vi "Untitled 1.vi"() -> ()   [LabVIEW 2020]
panel:
  in  "New Game":bool
  out "Turno":string
  in  "Ring 42":u16(ring)
  in  "Ring 41":u16(ring)
  in  "Ring 40":u16(ring)
  in  "Ring 39":u16(ring)
  in  "Ring 38":u16(ring)
  in  "Ring 37":u16(ring)
  in  "Ring 36":u16(ring)
  in  "Ring 35":u16(ring)
  in  "Ring 34":u16(ring)
  in  "Ring 33":u16(ring)
  in  "Ring 32":u16(ring)
  in  "Ring 31":u16(ring)
  in  "Ring 30":u16(ring)
  in  "Ring 29":u16(ring)
  in  "Ring 28":u16(ring)
  in  "Ring 27":u16(ring)
  in  "Ring 26":u16(ring)
  in  "Ring 25":u16(ring)
  in  "Ring 24":u16(ring)
  in  "Ring 23":u16(ring)
  in  "Ring 22":u16(ring)
  in  "Ring 21":u16(ring)
  in  "Ring 20":u16(ring)
  in  "Ring 19":u16(ring)
  in  "Ring 18":u16(ring)
  in  "Ring 17":u16(ring)
  in  "Ring 16":u16(ring)
  in  "Ring 15":u16(ring)
  in  "Ring 14":u16(ring)
  in  "Ring 13":u16(ring)
  in  "Ring 12":u16(ring)
  in  "Ring 11":u16(ring)
  in  "Ring 10":u16(ring)
  in  "Ring 9":u16(ring)
  in  "Ring 8":u16(ring)
  in  "Ring 7":u16(ring)
  in  "Ring 6":u16(ring)
  in  "Ring 5":u16(ring)
  in  "Ring 4":u16(ring)
  in  "Ring 3":u16(ring)
  in  "Ring 2":u16(ring)
  in  "Ring":u16(ring)
  # "CUATRO EN LINEA"
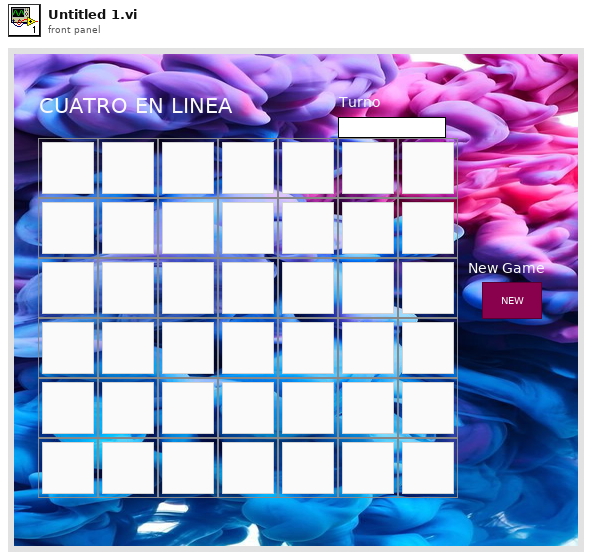
[diagram p1: front panel]
types:
  T1 = typedef "Symbol.ctl" = u16
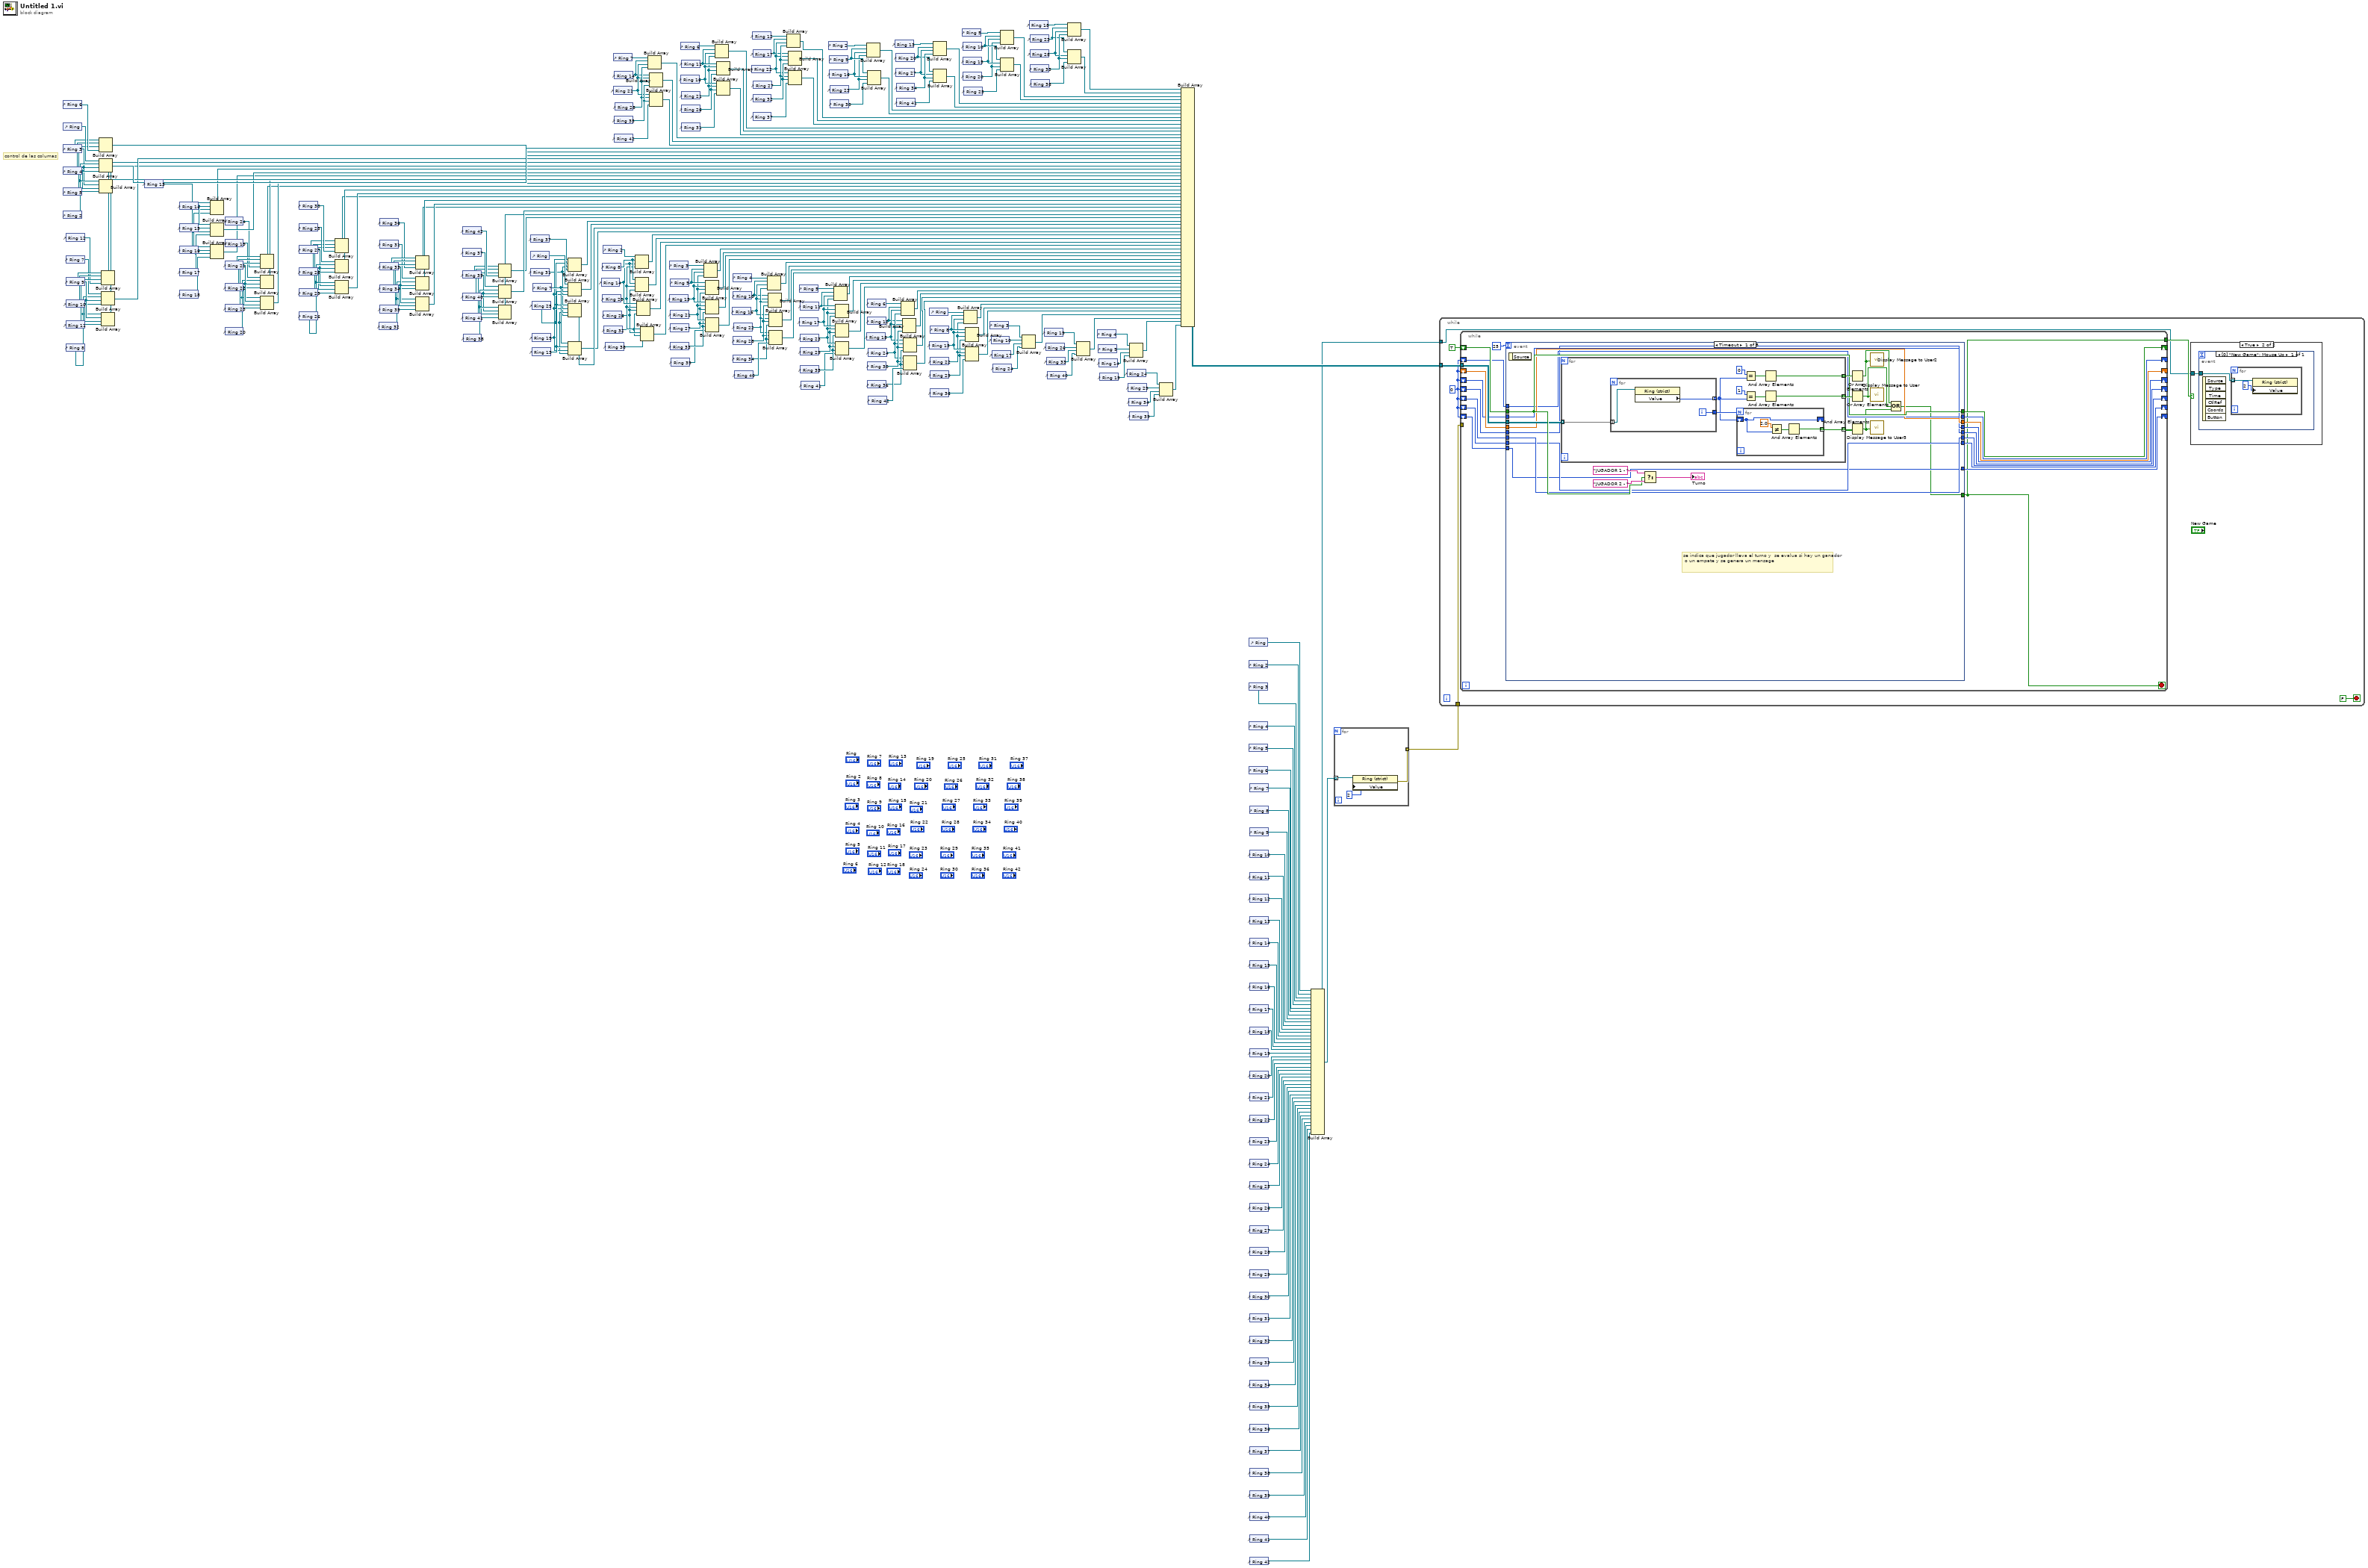
[diagram p0: block diagram]
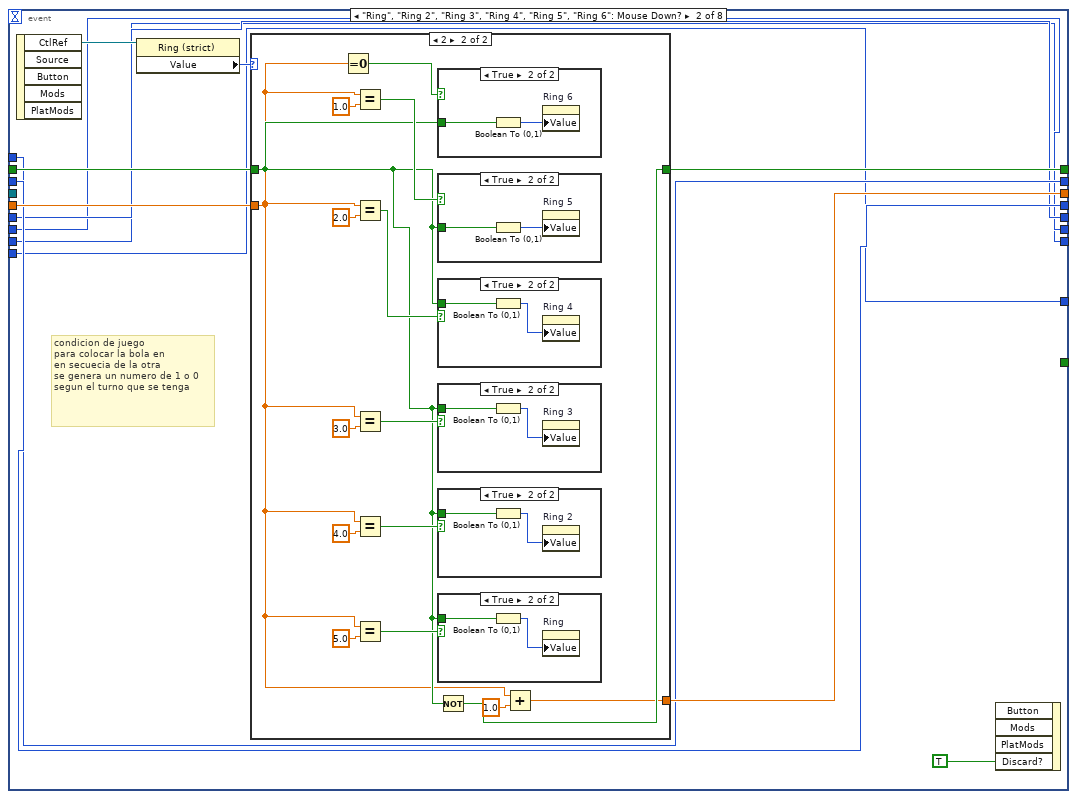
[diagram p3: hidden frame]
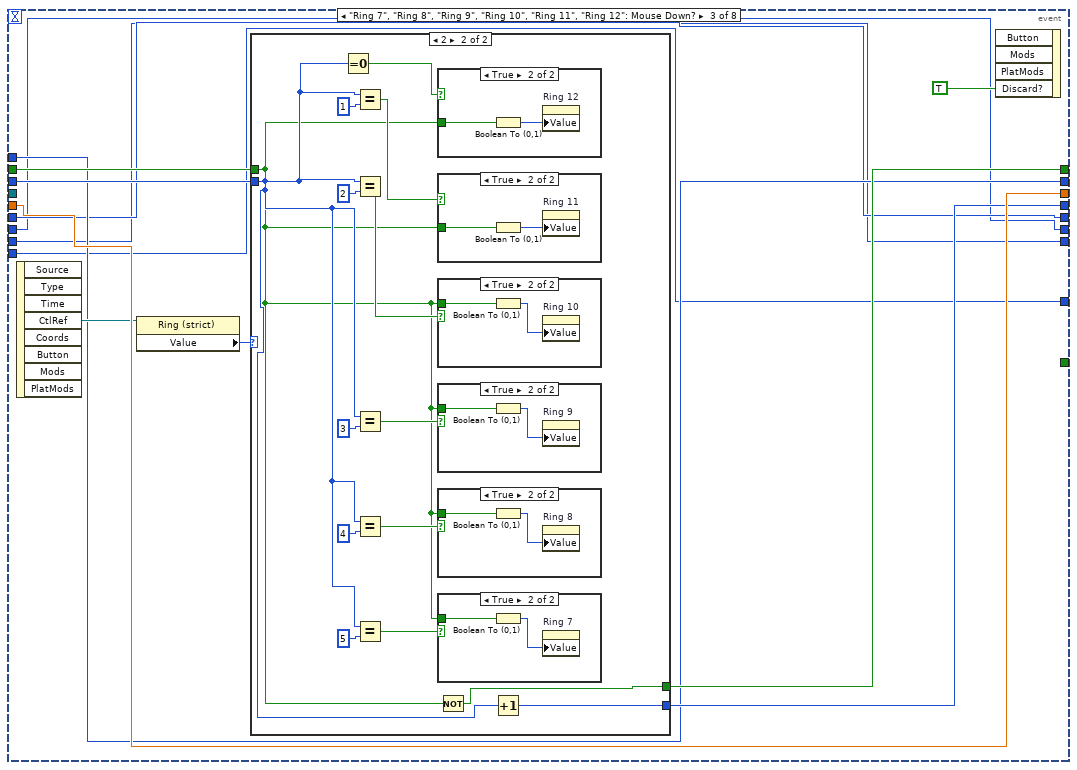
[diagram p11: hidden frame]
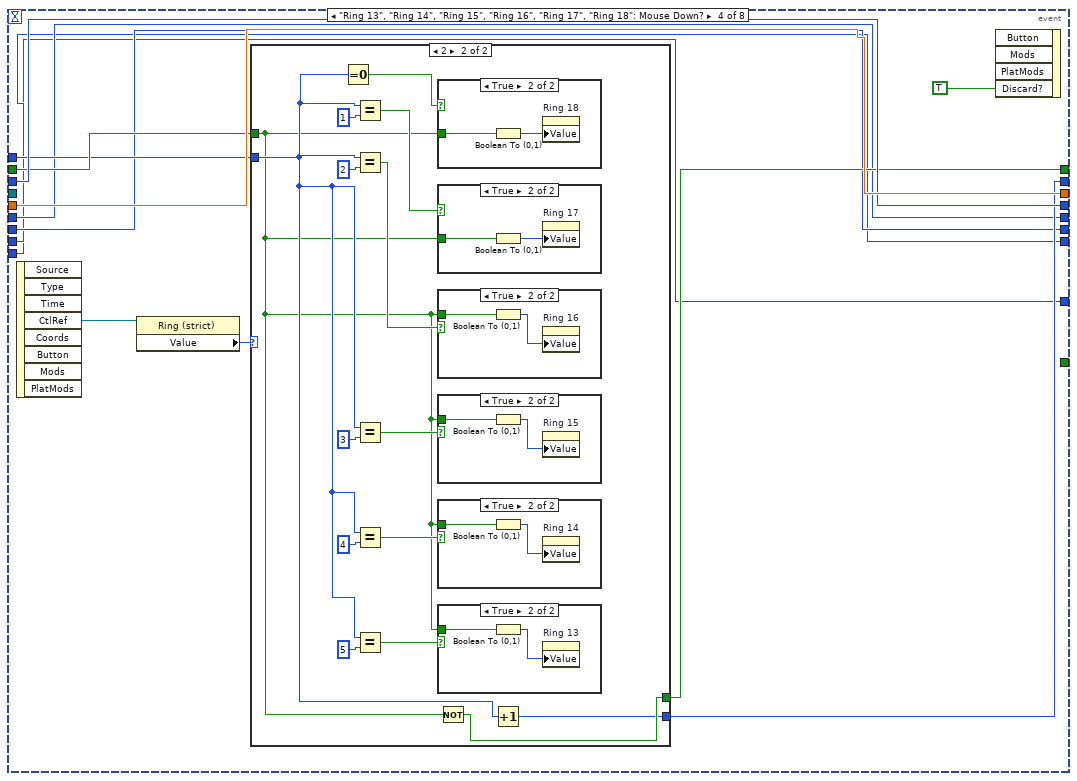
[diagram p19: hidden frame]
diagram:
  # "control de las columas"
  n1 = control-ref of="Ring 6"() -> (w213:refnum<vi>)
  n2 = control-ref of="Ring"() -> (w215:refnum<vi>)
  n3 = control-ref of="Ring 3"() -> (w210:refnum<vi>)
  n4 = control-ref of="Ring 4"() -> (w211:refnum<vi>)
  n5 = control-ref of="Ring 5"() -> (w212:refnum<vi>)
  n6 = control-ref of="Ring 2"() -> (w214:refnum<vi>)
  n7 = control-ref of="Ring 12"() -> (w206:refnum<vi>)
  n8 = control-ref of="Ring 7"() -> (w204:refnum<vi>)
  n9 = control-ref of="Ring 9"() -> (w209:refnum<vi>)
  n10 = control-ref of="Ring 10"() -> (w208:refnum<vi>)
  n11 = control-ref of="Ring 11"() -> (w207:refnum<vi>)
  n12 = control-ref of="Ring 8"() -> (w205:refnum<vi>)
  n13 = Build Array(w210, w211, w212, w213) -> (w201:refnum<vi>[])
  n14 = Build Array(w215, w214, w210, w211) -> (w203:refnum<vi>[])
  n15 = Build Array(w214, w210, w211, w212) -> (w202:refnum<vi>[])
  n16 = Build Array(w209, w208, w207, w206) -> (w198:refnum<vi>[])
  n17 = Build Array(w204, w205, w209, w208) -> (w200:refnum<vi>[])
  n18 = Build Array(w205, w209, w208, w207) -> (w199:refnum<vi>[])
  n19 = control-ref of="Ring 13"() -> (w196:refnum<vi>)
  n20 = control-ref of="Ring 14"() -> (w195:refnum<vi>)
  n21 = control-ref of="Ring 15"() -> (w191:refnum<vi>)
  n22 = control-ref of="Ring 16"() -> (w192:refnum<vi>)
  n23 = control-ref of="Ring 17"() -> (w193:refnum<vi>)
  n24 = control-ref of="Ring 18"() -> (w194:refnum<vi>)
  n25 = Build Array(w196, w195, w191, w192) -> (w190:refnum<vi>[])
  n26 = Build Array(w195, w191, w192, w193) -> (w189:refnum<vi>[])
  n27 = Build Array(w191, w192, w193, w194) -> (w188:refnum<vi>[])
  n28 = control-ref of="Ring 24"() -> (w184:refnum<vi>)
  n29 = control-ref of="Ring 19"() -> (w182:refnum<vi>)
  n30 = control-ref of="Ring 21"() -> (w187:refnum<vi>)
  n31 = control-ref of="Ring 22"() -> (w186:refnum<vi>)
  n32 = control-ref of="Ring 23"() -> (w185:refnum<vi>)
  n33 = control-ref of="Ring 20"() -> (w183:refnum<vi>)
  n34 = Build Array(w187, w186, w185, w184) -> (w179:refnum<vi>[])
  n35 = Build Array(w182, w183, w187, w186) -> (w181:refnum<vi>[])
  n36 = Build Array(w183, w187, w186, w185) -> (w180:refnum<vi>[])
  n37 = control-ref of="Ring 30"() -> (w176:refnum<vi>)
  n38 = control-ref of="Ring 25"() -> (w178:refnum<vi>)
  n39 = control-ref of="Ring 27"() -> (w173:refnum<vi>)
  n40 = control-ref of="Ring 28"() -> (w174:refnum<vi>)
  n41 = control-ref of="Ring 29"() -> (w175:refnum<vi>)
  n42 = control-ref of="Ring 26"() -> (w177:refnum<vi>)
  n43 = Build Array(w173, w174, w175, w176) -> (w170:refnum<vi>[])
  n44 = Build Array(w178, w177, w173, w174) -> (w172:refnum<vi>[])
  n45 = Build Array(w177, w173, w174, w175) -> (w171:refnum<vi>[])
  n46 = control-ref of="Ring 32"() -> (w165:refnum<vi>)
  n47 = control-ref of="Ring 36"() -> (w166:refnum<vi>)
  n48 = control-ref of="Ring 31"() -> (w164:refnum<vi>)
  n49 = control-ref of="Ring 33"() -> (w169:refnum<vi>)
  n50 = control-ref of="Ring 34"() -> (w168:refnum<vi>)
  n51 = control-ref of="Ring 35"() -> (w167:refnum<vi>)
  n52 = Build Array(w169, w168, w167, w166) -> (w161:refnum<vi>[])
  n53 = Build Array(w164, w165, w169, w168) -> (w163:refnum<vi>[])
  n54 = Build Array(w165, w169, w168, w167) -> (w162:refnum<vi>[])
  n55 = control-ref of="Ring 42"() -> (w158:refnum<vi>)
  n56 = control-ref of="Ring 37"() -> (w160:refnum<vi>)
  n57 = control-ref of="Ring 39"() -> (w155:refnum<vi>)
  n58 = control-ref of="Ring 40"() -> (w156:refnum<vi>)
  n59 = control-ref of="Ring 41"() -> (w157:refnum<vi>)
  n60 = control-ref of="Ring 38"() -> (w159:refnum<vi>)
  n61 = Build Array(w155, w156, w157, w158) -> (w152:refnum<vi>[])
  n62 = Build Array(w160, w159, w155, w156) -> (w154:refnum<vi>[])
  n63 = Build Array(w159, w155, w156, w157) -> (w153:refnum<vi>[])
  n64 = control-ref of="Ring 37"() -> (w145:refnum<vi>)
  n65 = control-ref of="Ring"() -> (w151:refnum<vi>)
  n66 = control-ref of="Ring 31"() -> (w146:refnum<vi>)
  n67 = control-ref of="Ring 25"() -> (w147:refnum<vi>)
  n68 = control-ref of="Ring 19"() -> (w148:refnum<vi>)
  n69 = control-ref of="Ring 13"() -> (w149:refnum<vi>)
  n70 = control-ref of="Ring 7"() -> (w150:refnum<vi>)
  n71 = Build Array(w148, w147, w146, w145) -> (w144:refnum<vi>[])
  n72 = Build Array(w151, w150, w149, w148) -> (w143:refnum<vi>[])
  n73 = Build Array(w149, w148, w147, w146) -> (w142:refnum<vi>[])
  n74 = Build Array(w150, w149, w148, w147) -> (w141:refnum<vi>[])
  n75 = control-ref of="Ring 14"() -> (w136:refnum<vi>)
  n76 = control-ref of="Ring 8"() -> (w138:refnum<vi>)
  n77 = control-ref of="Ring 20"() -> (w134:refnum<vi>)
  n78 = control-ref of="Ring 2"() -> (w140:refnum<vi>)
  n79 = control-ref of="Ring 26"() -> (w133:refnum<vi>)
  n80 = control-ref of="Ring 32"() -> (w132:refnum<vi>)
  n81 = control-ref of="Ring 38"() -> (w131:refnum<vi>)
  n82 = control-ref of="Ring 21"() -> (w73:refnum<vi>)
  n83 = control-ref of="Ring 7"() -> (w71:refnum<vi>)
  n84 = control-ref of="Ring 14"() -> (w72:refnum<vi>)
  n85 = control-ref of="Ring 35"() -> (w75:refnum<vi>)
  n86 = control-ref of="Ring 42"() -> (w76:refnum<vi>)
  n87 = control-ref of="Ring 28"() -> (w74:refnum<vi>)
  n88 = Build Array(w140, w138, w136, w134) -> (w139:refnum<vi>[])
  n89 = Build Array(w138, w136, w134, w133) -> (w137:refnum<vi>[])
  n90 = Build Array(w136, w134, w133, w132) -> (w135:refnum<vi>[])
  n91 = Build Array(w134, w133, w132, w131) -> (w130:refnum<vi>[])
  n92 = Build Array(w71, w72, w73, w74) -> (w68:refnum<vi>[])
  n93 = Build Array(w72, w73, w74, w75) -> (w69:refnum<vi>[])
  n94 = Build Array(w73, w74, w75, w76) -> (w70:refnum<vi>[])
  n95 = control-ref of="Ring 15"() -> (w125:refnum<vi>)
  n96 = control-ref of="Ring 3"() -> (w129:refnum<vi>)
  n97 = control-ref of="Ring 9"() -> (w127:refnum<vi>)
  n98 = control-ref of="Ring 27"() -> (w122:refnum<vi>)
  n99 = control-ref of="Ring 33"() -> (w121:refnum<vi>)
  n100 = control-ref of="Ring 21"() -> (w123:refnum<vi>)
  n101 = control-ref of="Ring 39"() -> (w120:refnum<vi>)
  n102 = control-ref of="Ring 16"() -> (w65:refnum<vi>)
  n103 = control-ref of="Ring 6"() -> (w67:refnum<vi>)
  n104 = control-ref of="Ring 11"() -> (w66:refnum<vi>)
  n105 = control-ref of="Ring 26"() -> (w63:refnum<vi>)
  n106 = control-ref of="Ring 31"() -> (w62:refnum<vi>)
  n107 = control-ref of="Ring 21"() -> (w64:refnum<vi>)
  n108 = Build Array(w129, w127, w125, w123) -> (w128:refnum<vi>[])
  n109 = Build Array(w127, w125, w123, w122) -> (w126:refnum<vi>[])
  n110 = Build Array(w125, w123, w122, w121) -> (w124:refnum<vi>[])
  n111 = Build Array(w123, w122, w121, w120) -> (w119:refnum<vi>[])
  n112 = Build Array(w67, w66, w65, w64) -> (w59:refnum<vi>[])
  n113 = Build Array(w66, w65, w64, w63) -> (w60:refnum<vi>[])
  n114 = Build Array(w65, w64, w63, w62) -> (w61:refnum<vi>[])
  n115 = control-ref of="Ring 16"() -> (w114:refnum<vi>)
  n116 = control-ref of="Ring 4"() -> (w112:refnum<vi>)
  n117 = control-ref of="Ring 10"() -> (w113:refnum<vi>)
  n118 = control-ref of="Ring 28"() -> (w116:refnum<vi>)
  n119 = control-ref of="Ring 34"() -> (w117:refnum<vi>)
  n120 = control-ref of="Ring 22"() -> (w115:refnum<vi>)
  n121 = control-ref of="Ring 40"() -> (w118:refnum<vi>)
  n122 = control-ref of="Ring 22"() -> (w55:refnum<vi>)
  n123 = control-ref of="Ring 12"() -> (w53:refnum<vi>)
  n124 = control-ref of="Ring 17"() -> (w54:refnum<vi>)
  n125 = control-ref of="Ring 32"() -> (w57:refnum<vi>)
  n126 = control-ref of="Ring 37"() -> (w58:refnum<vi>)
  n127 = control-ref of="Ring 27"() -> (w56:refnum<vi>)
  n128 = Build Array(w112, w113, w114, w115) -> (w111:refnum<vi>[])
  n129 = Build Array(w113, w114, w115, w116) -> (w110:refnum<vi>[])
  n130 = Build Array(w114, w115, w116, w117) -> (w109:refnum<vi>[])
  n131 = Build Array(w115, w116, w117, w118) -> (w108:refnum<vi>[])
  n132 = Build Array(w53, w54, w55, w56) -> (w50:refnum<vi>[])
  n133 = Build Array(w54, w55, w56, w57) -> (w51:refnum<vi>[])
  n134 = Build Array(w55, w56, w57, w58) -> (w52:refnum<vi>[])
  n135 = control-ref of="Ring 17"() -> (w105:refnum<vi>)
  n136 = control-ref of="Ring 5"() -> (w107:refnum<vi>)
  n137 = control-ref of="Ring 11"() -> (w106:refnum<vi>)
  n138 = control-ref of="Ring 29"() -> (w103:refnum<vi>)
  n139 = control-ref of="Ring 35"() -> (w102:refnum<vi>)
  n140 = control-ref of="Ring 23"() -> (w104:refnum<vi>)
  n141 = control-ref of="Ring 41"() -> (w101:refnum<vi>)
  n142 = control-ref of="Ring 2"() -> (w49:refnum<vi>)
  n143 = control-ref of="Ring 9"() -> (w48:refnum<vi>)
  n144 = control-ref of="Ring 16"() -> (w47:refnum<vi>)
  n145 = control-ref of="Ring 23"() -> (w46:refnum<vi>)
  n146 = control-ref of="Ring 30"() -> (w45:refnum<vi>)
  n147 = Build Array(w107, w106, w105, w104) -> (w100:refnum<vi>[])
  n148 = Build Array(w106, w105, w104, w103) -> (w99:refnum<vi>[])
  n149 = Build Array(w105, w104, w103, w102) -> (w98:refnum<vi>[])
  n150 = Build Array(w104, w103, w102, w101) -> (w97:refnum<vi>[])
  n151 = Build Array(w49, w48, w47, w46) -> (w43:refnum<vi>[])
  n152 = control-ref of="Ring 18"() -> (w92:refnum<vi>)
  n153 = Build Array(w48, w47, w46, w45) -> (w44:refnum<vi>[])
  n154 = control-ref of="Ring 6"() -> (w90:refnum<vi>)
  n155 = control-ref of="Ring 12"() -> (w91:refnum<vi>)
  n156 = control-ref of="Ring 30"() -> (w94:refnum<vi>)
  n157 = control-ref of="Ring 36"() -> (w95:refnum<vi>)
  n158 = control-ref of="Ring 24"() -> (w93:refnum<vi>)
  n159 = control-ref of="Ring 42"() -> (w96:refnum<vi>)
  n160 = control-ref of="Ring 13"() -> (w38:refnum<vi>)
  n161 = control-ref of="Ring 20"() -> (w39:refnum<vi>)
  n162 = control-ref of="Ring 27"() -> (w40:refnum<vi>)
  n163 = control-ref of="Ring 34"() -> (w41:refnum<vi>)
  n164 = control-ref of="Ring 41"() -> (w42:refnum<vi>)
  n165 = Build Array(w90, w91, w92, w93) -> (w89:refnum<vi>[])
  n166 = Build Array(w91, w92, w93, w94) -> (w88:refnum<vi>[])
  n167 = Build Array(w92, w93, w94, w95) -> (w87:refnum<vi>[])
  n168 = Build Array(w93, w94, w95, w96) -> (w86:refnum<vi>[])
  n169 = control-ref of="Ring 15"() -> (w83:refnum<vi>)
  n170 = control-ref of="Ring"() -> (w85:refnum<vi>)
  n171 = control-ref of="Ring 8"() -> (w84:refnum<vi>)
  n172 = control-ref of="Ring 29"() -> (w81:refnum<vi>)
  n173 = control-ref of="Ring 36"() -> (w80:refnum<vi>)
  n174 = control-ref of="Ring 22"() -> (w82:refnum<vi>)
  n175 = Build Array(w38, w39, w40, w41) -> (w36:refnum<vi>[])
  n176 = Build Array(w39, w40, w41, w42) -> (w37:refnum<vi>[])
  n177 = control-ref of="Ring 5"() -> (w35:refnum<vi>)
  n178 = control-ref of="Ring 10"() -> (w34:refnum<vi>)
  n179 = control-ref of="Ring 15"() -> (w33:refnum<vi>)
  n180 = control-ref of="Ring 20"() -> (w32:refnum<vi>)
  n181 = control-ref of="Ring 25"() -> (w31:refnum<vi>)
  n182 = Build Array(w85, w84, w83, w82) -> (w79:refnum<vi>[])
  n183 = Build Array(w84, w83, w82, w81) -> (w78:refnum<vi>[])
  n184 = Build Array(w83, w82, w81, w80) -> (w77:refnum<vi>[])
  n185 = control-ref of="Ring 3"() -> (w21:refnum<vi>)
  n186 = control-ref of="Ring 10"() -> (w20:refnum<vi>)
  n187 = control-ref of="Ring 17"() -> (w19:refnum<vi>)
  n188 = control-ref of="Ring 24"() -> (w18:refnum<vi>)
  n189 = Build Array(w35, w34, w33, w32) -> (w29:refnum<vi>[])
  n190 = Build Array(w34, w33, w32, w31) -> (w30:refnum<vi>[])
  n191 = Build Array(w21, w20, w19, w18) -> (w17:refnum<vi>[])
  n192 = control-ref of="Ring 18"() -> (w24:refnum<vi>)
  n193 = control-ref of="Ring 23"() -> (w25:refnum<vi>)
  n194 = control-ref of="Ring 28"() -> (w26:refnum<vi>)
  n195 = control-ref of="Ring 33"() -> (w27:refnum<vi>)
  n196 = control-ref of="Ring 38"() -> (w28:refnum<vi>)
  n197 = control-ref of="Ring 19"() -> (w13:refnum<vi>)
  n198 = control-ref of="Ring 26"() -> (w14:refnum<vi>)
  n199 = control-ref of="Ring 33"() -> (w15:refnum<vi>)
  n200 = control-ref of="Ring 40"() -> (w16:refnum<vi>)
  n201 = Build Array(w24, w25, w26, w27) -> (w22:refnum<vi>[])
  n202 = Build Array(w25, w26, w27, w28) -> (w23:refnum<vi>[])
  n203 = Build Array(w13, w14, w15, w16) -> (w12:refnum<vi>[])
  n204 = control-ref of="Ring 4"() -> (w11:refnum<vi>)
  n205 = control-ref of="Ring 9"() -> (w10:refnum<vi>)
  n206 = control-ref of="Ring 14"() -> (w9:refnum<vi>)
  n207 = control-ref of="Ring 19"() -> (w8:refnum<vi>)
  n208 = control-ref of="Ring 24"() -> (w3:refnum<vi>)
  n209 = control-ref of="Ring 29"() -> (w4:refnum<vi>)
  n210 = control-ref of="Ring 34"() -> (w5:refnum<vi>)
  n211 = Build Array(w11, w10, w9, w8) -> (w7:refnum<vi>[])
  n212 = control-ref of="Ring 39"() -> (w6:refnum<vi>)
  n213 = Build Array(w3, w4, w5, w6) -> (w2:refnum<vi>[])
  n214 = Build Array(w22, w23, w29, w30, w36, w37, w43, w44, w50, w51, w52, w59, w60, w61, w68, w69, w70, w203, w202, w201, w200, w199, w198, w190, w189, w188, w181, w180, w179, w172, w171, w170, w163, w162, w161, w154, w153, w152, w144, w143, w142, w141, w139, w137, w135, w130, w128, w126, w124, w119, w111, w110, w109, w108, w100, w99, w98, w97, w89, w88, w87, w86, w79, w78, w77, w17, w12, w7, w2) -> (w197:refnum<vi>[][])
  n215 = control-ref of="Ring"() -> (w258:refnum<vi>)
  n216 = control-ref of="Ring 2"() -> (w257:refnum<vi>)
  n217 = control-ref of="Ring 3"() -> (w256:refnum<vi>)
  n218 = control-ref of="Ring 4"() -> (w255:refnum<vi>)
  n219 = control-ref of="Ring 5"() -> (w254:refnum<vi>)
  n220 = control-ref of="Ring 6"() -> (w253:refnum<vi>)
  n221 = control-ref of="Ring 7"() -> (w252:refnum<vi>)
  n222 = control-ref of="Ring 8"() -> (w251:refnum<vi>)
  n223 = control-ref of="Ring 9"() -> (w250:refnum<vi>)
  n224 = control-ref of="Ring 10"() -> (w249:refnum<vi>)
  n225 = control-ref of="Ring 11"() -> (w248:refnum<vi>)
  n226 = control-ref of="Ring 12"() -> (w247:refnum<vi>)
  n227 = control-ref of="Ring 13"() -> (w246:refnum<vi>)
  n228 = control-ref of="Ring 14"() -> (w245:refnum<vi>)
  n229 = control-ref of="Ring 15"() -> (w244:refnum<vi>)
  n230 = control-ref of="Ring 16"() -> (w243:refnum<vi>)
  n231 = control-ref of="Ring 17"() -> (w242:refnum<vi>)
  n232 = control-ref of="Ring 18"() -> (w241:refnum<vi>)
  n233 = control-ref of="Ring 19"() -> (w240:refnum<vi>)
  n234 = control-ref of="Ring 20"() -> (w239:refnum<vi>)
  n235 = control-ref of="Ring 21"() -> (w238:refnum<vi>)
  n236 = control-ref of="Ring 22"() -> (w237:refnum<vi>)
  n237 = control-ref of="Ring 23"() -> (w236:refnum<vi>)
  n238 = control-ref of="Ring 24"() -> (w235:refnum<vi>)
  n239 = control-ref of="Ring 25"() -> (w234:refnum<vi>)
  n240 = control-ref of="Ring 26"() -> (w233:refnum<vi>)
  n241 = control-ref of="Ring 27"() -> (w232:refnum<vi>)
  n242 = control-ref of="Ring 28"() -> (w231:refnum<vi>)
  n243 = control-ref of="Ring 29"() -> (w230:refnum<vi>)
  n244 = control-ref of="Ring 30"() -> (w229:refnum<vi>)
  n245 = control-ref of="Ring 31"() -> (w228:refnum<vi>)
  n246 = control-ref of="Ring 32"() -> (w227:refnum<vi>)
  n247 = control-ref of="Ring 33"() -> (w226:refnum<vi>)
  n248 = control-ref of="Ring 34"() -> (w225:refnum<vi>)
  n249 = control-ref of="Ring 35"() -> (w224:refnum<vi>)
  n250 = control-ref of="Ring 36"() -> (w223:refnum<vi>)
  n251 = control-ref of="Ring 37"() -> (w222:refnum<vi>)
  n252 = control-ref of="Ring 38"() -> (w221:refnum<vi>)
  n253 = control-ref of="Ring 39"() -> (w220:refnum<vi>)
  n254 = control-ref of="Ring 40"() -> (w219:refnum<vi>)
  n255 = control-ref of="Ring 41"() -> (w218:refnum<vi>)
  n256 = control-ref of="Ring 42"() -> (w217:refnum<vi>)
  n257 = Build Array(w258, w257, w256, w255, w254, w253, w252, w251, w250, w249, w248, w247, w246, w245, w244, w243, w242, w241, w240, w239, w238, w237, w236, w235, w234, w233, w232, w231, w230, w229, w228, w227, w226, w225, w224, w223, w222, w221, w220, w219, w218, w217) -> (w1:refnum<vi>[])
  n258 = for {
    tunnel: w1 -> [w261] mode=indexing
    tunnel: [w259] -> w216 mode=indexing
    n259 = property class="Ring (strict)"(reference=w261, "Value"=u16 2) -> (error out=w259:errorcluster)  [unwired: 1 in, 1 out]
  }
  n260 = while {
    tunnel: w216 -> [w268]
    tunnel: w197 -> [w267]
    tunnel: w1 -> [w263]
    stop <- FALSE stop-if-true
    w265 = 0
    n261 = while {
      tunnel: w268 -> [_]
      tunnel: w267 -> [w288]
      shift-right: [w289] -> _
      shift-left: TRUE -> [w290]
      shift-right: [w286] -> _
      shift-left: w265 -> [w287]
      shift-right: [w284] -> _
      shift-left: w265 -> [w285]
      shift-right: [w282] -> _
      shift-left: w265 -> [w283]
      shift-right: [w280] -> _
      shift-left: w265 -> [w281]
      shift-right: [w278] -> _
      shift-left: w265 -> [w279]
      shift-right: [w276] -> _
      shift-left: w265 -> [w277]
      shift-right: [w274] -> _
      shift-left: w265 -> [w275]
      tunnel: [w273] -> w264
      stop <- w273 stop-if-true
      n262 = event shown="[0] Timeout" {
        selector: _ -> [_ _ _ _ _ _ _ _]
        dyn-events: _ -> [_ _ _ _ _ _ _ _]
        timeout: 25 -> [_ _ _ _ _ _ _ _]
        tunnel: [w303 w340 w378 w417 w454 w492 w531 w570] -> w289
        tunnel: [w292 _ _ _ _ _ _ _] -> w273
        tunnel: w290 -> [w303 w338 w379 w418 w455 w493 w532 w571]
        tunnel: w288 -> [w302 _ _ _ _ _ _ _]
        tunnel: w287 -> [w301 w335 w382 w420 w460 w499 w541 w579]
        tunnel: [w301 w334 w382 w420 w460 w499 w541 w579] -> w286
        tunnel: w285 -> [w300 w333 w377 w419 w459 w498 w540 w578]
        tunnel: [w300 w333 w376 w419 w459 w498 w540 w578] -> w284
        tunnel: w283 -> [w299 w332 w374 w415 w461 w500 w542 w580]
        tunnel: [w299 w332 w374 w414 w461 w500 w542 w580] -> w282
        tunnel: w281 -> [w298 w331 w373 w413 w457 w497 w539 w577]
        tunnel: [w298 w331 w373 w413 w456 w497 w539 w577] -> w280
        tunnel: w279 -> [w297 w330 w372 w412 w452 w495 w538 w576]
        tunnel: [w297 w330 w372 w412 w452 w494 w538 w576] -> w278
        tunnel: w277 -> [w296 w329 w371 w411 w451 w491 w534 w575]
        tunnel: [w296 w329 w371 w411 w451 w491 w533 w575] -> w276
        tunnel: w275 -> [w295 w328 w370 w410 w450 w490 w530 w573]
        tunnel: [w295 w328 w370 w410 w450 w490 w530 w572] -> w274
        event Timeout {
          # "se indica que jugador lleva el turno y  se evalua si hay un ganador\n o un empate y se genera un mensage"
          n263 = event-data() -> ()  [unwired: 1 in, 1 out]
          n264 = for {
            tunnel: [w318] -> w306 mode=indexing
            tunnel: [w317] -> w307 mode=indexing
            tunnel: w302 -> [w316] mode=indexing
            tunnel: [w311] -> w294 mode=indexing
            n265 = for {
              tunnel: [w327] -> w312 mode=indexing
              tunnel: w316 -> [w326] mode=indexing
              tunnel: [w325] -> w313
              i -> [w325]
              n266 = property class="Ring (strict)"(reference=w326) -> ("Value"=w327:T1)  [unwired: 1 in, 2 out]
            }
            n267 = for {
              N: w313 -> [_]
              shift-right: [w322] -> _
              shift-left: w312 -> [w322]
              tunnel: [w321] -> w311 mode=indexing
              n268 = Not Equal?(x=2.0, y=w322) -> (x != y?=w323:bool[])
              n269 = And Array Elements(Boolean array=w323) -> (logical AND=w321:bool)
            }
            n270 = Equal?(x=0, y=w312) -> (x = y?=w320:bool[])
            n271 = Equal?(x=1, y=w312) -> (x = y?=w319:bool[])
            n272 = And Array Elements(Boolean array=w320) -> (logical AND=w317:bool)
            n273 = And Array Elements(Boolean array=w319) -> (logical AND=w318:bool)
          }
          n274 = Select(t="JUGADOR 1 - ", s=w303, f="JUGADOR 2 - ") -> (s? t:f=→"Turno":string)
          n275 = Or Array Elements(Boolean array=w307) -> (logical OR=w305:bool)
          n276 = Or Array Elements(Boolean array=w306) -> (logical OR=w304:bool)
          n277 = And Array Elements(Boolean array=w294) -> (logical AND=w293:bool)
          n278 = call "Display Message to User2"("Enable"=w305) -> ()  [unwired: 9 in, 2 out]
          n279 = call "Display Message to User"("Enable"=w304) -> ()  [unwired: 9 in, 2 out]
          n280 = call "Display Message to User3"("Enable"=w293) -> ()  [unwired: 9 in, 2 out]
          n281 = Compound Arithmetic op=OR(w305, w304, w293) -> (w292:bool)
        }
        event "Ring", "Ring 2", "Ring 3", "Ring 4", "Ring 5", "Ring 6": Mouse Down? {
          # "condicion de juego \npara colocar la bola en \nen secuecia de la otra \nse genera un numero de 1 o 0 \nsegun el turno que se tenga"
          n282 = event-data() -> ("CtlRef"=w337:refnum<vi>)  [unwired: 1 in, 4 out]
          n283 = property class="Ring (strict)"(reference=w337) -> ("Value"=w336:u16)  [unwired: 1 in, 2 out]
          n284 = case shown="2" w336 {
            tunnel: [w341 w357] -> w340
            tunnel: w338 -> [w341 w343]
            tunnel: w335 -> [_ w342]
            tunnel: [_ w356] -> w334
            frame Default {
              # "DO not touch the values here"
            }
            frame 2 {
              n285 = Equal To 0?(x=w342) -> (x = 0?=w354:bool)
              n286 = Equal?(x=w342, y=1.0) -> (x = y?=w353:bool)
              n287 = Equal?(x=w342, y=2.0) -> (x = y?=w350:bool)
              n288 = Equal?(x=w342, y=3.0) -> (x = y?=w349:bool)
              n289 = Equal?(x=w342, y=4.0) -> (x = y?=w346:bool)
              n290 = Equal?(x=w342, y=5.0) -> (x = y?=w345:bool)
              n291 = case shown="True" w354 {
                tunnel: w343 -> [_ w368]
                frame False {
                }
                frame True {
                  n292 = Boolean To (0,1)(Boolean=w368) -> (0, 1=w369:i16)
                  n293 = property on="Ring 6" class="Ring (strict)"("Value"=w369) -> ()  [unwired: 2 in, 2 out]
                }
              }
              n294 = case shown="True" w353 {
                tunnel: w343 -> [_ w366]
                frame False {
                }
                frame True {
                  n295 = Boolean To (0,1)(Boolean=w366) -> (0, 1=w367:i16)
                  n296 = property on="Ring 5" class="Ring (strict)"("Value"=w367) -> ()  [unwired: 2 in, 2 out]
                }
              }
              n297 = case shown="True" w350 {
                tunnel: w343 -> [_ w364]
                frame False {
                }
                frame True {
                  n298 = Boolean To (0,1)(Boolean=w364) -> (0, 1=w365:i16)
                  n299 = property on="Ring 4" class="Ring (strict)"("Value"=w365) -> ()  [unwired: 2 in, 2 out]
                }
              }
              n300 = case shown="True" w349 {
                tunnel: w343 -> [_ w362]
                frame False {
                }
                frame True {
                  n301 = Boolean To (0,1)(Boolean=w362) -> (0, 1=w363:i16)
                  n302 = property on="Ring 3" class="Ring (strict)"("Value"=w363) -> ()  [unwired: 2 in, 2 out]
                }
              }
              n303 = case shown="True" w346 {
                tunnel: w343 -> [_ w360]
                frame False {
                }
                frame True {
                  n304 = Boolean To (0,1)(Boolean=w360) -> (0, 1=w361:i16)
                  n305 = property on="Ring 2" class="Ring (strict)"("Value"=w361) -> ()  [unwired: 2 in, 2 out]
                }
              }
              n306 = case shown="True" w345 {
                tunnel: w343 -> [_ w358]
                frame False {
                }
                frame True {
                  n307 = Boolean To (0,1)(Boolean=w358) -> (0, 1=w359:i16)
                  n308 = property on="Ring" class="Ring (strict)"("Value"=w359) -> ()  [unwired: 2 in, 2 out]
                }
              }
              n309 = Not(x=w343) -> (.not. x?=w357:bool)
              n310 = Add(x=w342, y=1.0) -> (x+y=w356:dbl)
            }
          }
          n311 = event-data("Discard?"=TRUE) -> ()  [unwired: 4 in, 1 out]
        }
        event "Ring 7", "Ring 8", "Ring 9", "Ring 10", "Ring 11", "Ring 12": Mouse Down? {
          n312 = event-data() -> ("CtlRef"=w381:refnum<vi>)  [unwired: 1 in, 7 out]
          n313 = property class="Ring (strict)"(reference=w381) -> ("Value"=w380:u16)  [unwired: 1 in, 2 out]
          n314 = case shown="2" w380 {
            tunnel: w379 -> [_ w384]
            tunnel: [_ w383] -> w378
            tunnel: w377 -> [_ w386]
            tunnel: [_ w397] -> w376
            frame Default {
            }
            frame 2 {
              n315 = Equal To 0?(x=w386) -> (x = 0?=w396:bool)
              n316 = Equal?(x=w386, y=1) -> (x = y?=w395:bool)
              n317 = Equal?(x=w386, y=2) -> (x = y?=w392:bool)
              n318 = Equal?(x=w386, y=3) -> (x = y?=w390:bool)
              n319 = Equal?(x=w386, y=4) -> (x = y?=w388:bool)
              n320 = Equal?(x=w386, y=5) -> (x = y?=w385:bool)
              n321 = case shown="True" w396 {
                tunnel: w384 -> [_ w408]
                frame False {
                }
                frame True {
                  n322 = Boolean To (0,1)(Boolean=w408) -> (0, 1=w409:i16)
                  n323 = property on="Ring 12" class="Ring (strict)"("Value"=w409) -> ()  [unwired: 2 in, 2 out]
                }
              }
              n324 = case shown="True" w395 {
                tunnel: w384 -> [_ w406]
                frame False {
                }
                frame True {
                  n325 = Boolean To (0,1)(Boolean=w406) -> (0, 1=w407:i16)
                  n326 = property on="Ring 11" class="Ring (strict)"("Value"=w407) -> ()  [unwired: 2 in, 2 out]
                }
              }
              n327 = case shown="True" w392 {
                tunnel: w384 -> [_ w404]
                frame False {
                }
                frame True {
                  n328 = Boolean To (0,1)(Boolean=w404) -> (0, 1=w405:i16)
                  n329 = property on="Ring 10" class="Ring (strict)"("Value"=w405) -> ()  [unwired: 2 in, 2 out]
                }
              }
              n330 = case shown="True" w390 {
                tunnel: w384 -> [_ w402]
                frame False {
                }
                frame True {
                  n331 = Boolean To (0,1)(Boolean=w402) -> (0, 1=w403:i16)
                  n332 = property on="Ring 9" class="Ring (strict)"("Value"=w403) -> ()  [unwired: 2 in, 2 out]
                }
              }
              n333 = case shown="True" w388 {
                tunnel: w384 -> [_ w400]
                frame False {
                }
                frame True {
                  n334 = Boolean To (0,1)(Boolean=w400) -> (0, 1=w401:i16)
                  n335 = property on="Ring 8" class="Ring (strict)"("Value"=w401) -> ()  [unwired: 2 in, 2 out]
                }
              }
              n336 = case shown="True" w385 {
                tunnel: w384 -> [_ w398]
                frame False {
                }
                frame True {
                  n337 = Boolean To (0,1)(Boolean=w398) -> (0, 1=w399:i16)
                  n338 = property on="Ring 7" class="Ring (strict)"("Value"=w399) -> ()  [unwired: 2 in, 2 out]
                }
              }
              n339 = Not(x=w384) -> (.not. x?=w383:bool)
              n340 = Increment(x=w386) -> (x+1=w397:i32)
            }
          }
          n341 = event-data("Discard?"=TRUE) -> ()  [unwired: 4 in, 1 out]
        }
        event "Ring 13", "Ring 14", "Ring 15", "Ring 16", "Ring 17", "Ring 18": Mouse Down? {
          n342 = event-data() -> ("CtlRef"=w421:refnum<vi>)  [unwired: 1 in, 7 out]
          n343 = property class="Ring (strict)"(reference=w421) -> ("Value"=w416:u16)  [unwired: 1 in, 2 out]
          n344 = case shown="2" w416 {
            tunnel: w418 -> [_ w423]
            tunnel: [_ w437] -> w417
            tunnel: w415 -> [_ w425]
            tunnel: [_ w424] -> w414
            frame Default {
            }
            frame 2 {
              n345 = Equal To 0?(x=w425) -> (x = 0?=w436:bool)
              n346 = Equal?(x=w425, y=1) -> (x = y?=w435:bool)
              n347 = Equal?(x=w425, y=2) -> (x = y?=w429:bool)
              n348 = Equal?(x=w425, y=3) -> (x = y?=w428:bool)
              n349 = Equal?(x=w425, y=4) -> (x = y?=w427:bool)
              n350 = Equal?(x=w425, y=5) -> (x = y?=w426:bool)
              n351 = case shown="True" w436 {
                tunnel: w423 -> [_ w448]
                frame False {
                }
                frame True {
                  n352 = Boolean To (0,1)(Boolean=w448) -> (0, 1=w449:i16)
                  n353 = property on="Ring 18" class="Ring (strict)"("Value"=w449) -> ()  [unwired: 2 in, 2 out]
                }
              }
              n354 = case shown="True" w435 {
                tunnel: w423 -> [_ w446]
                frame False {
                }
                frame True {
                  n355 = Boolean To (0,1)(Boolean=w446) -> (0, 1=w447:i16)
                  n356 = property on="Ring 17" class="Ring (strict)"("Value"=w447) -> ()  [unwired: 2 in, 2 out]
                }
              }
              n357 = case shown="True" w429 {
                tunnel: w423 -> [_ w444]
                frame False {
                }
                frame True {
                  n358 = Boolean To (0,1)(Boolean=w444) -> (0, 1=w445:i16)
                  n359 = property on="Ring 16" class="Ring (strict)"("Value"=w445) -> ()  [unwired: 2 in, 2 out]
                }
              }
              n360 = case shown="True" w428 {
                tunnel: w423 -> [_ w442]
                frame False {
                }
                frame True {
                  n361 = Boolean To (0,1)(Boolean=w442) -> (0, 1=w443:i16)
                  n362 = property on="Ring 15" class="Ring (strict)"("Value"=w443) -> ()  [unwired: 2 in, 2 out]
                }
              }
              n363 = case shown="True" w427 {
                tunnel: w423 -> [_ w440]
                frame False {
                }
                frame True {
                  n364 = Boolean To (0,1)(Boolean=w440) -> (0, 1=w441:i16)
                  n365 = property on="Ring 14" class="Ring (strict)"("Value"=w441) -> ()  [unwired: 2 in, 2 out]
                }
              }
              n366 = case shown="True" w426 {
                tunnel: w423 -> [_ w438]
                frame False {
                }
                frame True {
                  n367 = Boolean To (0,1)(Boolean=w438) -> (0, 1=w439:i16)
                  n368 = property on="Ring 13" class="Ring (strict)"("Value"=w439) -> ()  [unwired: 2 in, 2 out]
                }
              }
              n369 = Not(x=w423) -> (.not. x?=w437:bool)
              n370 = Increment(x=w425) -> (x+1=w424:i32)
            }
          }
          n371 = event-data("Discard?"=TRUE) -> ()  [unwired: 4 in, 1 out]
        }
        event "Ring 19", "Ring 20", "Ring 21", "Ring 22", "Ring 23", "Ring 24": Mouse Down? {
          n372 = event-data() -> ("CtlRef"=w462:refnum<vi>)  [unwired: 1 in, 7 out]
          n373 = property class="Ring (strict)"(reference=w462) -> ("Value"=w458:u16)  [unwired: 1 in, 2 out]
          n374 = case shown="2" w458 {
            tunnel: w457 -> [_ w464]
            tunnel: [_ w477] -> w456
            tunnel: w455 -> [_ w474]
            tunnel: [_ w475] -> w454
            frame Default {
            }
            frame 2 {
              n375 = Equal To 0?(x=w464) -> (x = 0?=w476:bool)
              n376 = Equal?(x=w464, y=1) -> (x = y?=w472:bool)
              n377 = Equal?(x=w464, y=2) -> (x = y?=w467:bool)
              n378 = Equal?(x=w464, y=3) -> (x = y?=w466:bool)
              n379 = Equal?(x=w464, y=4) -> (x = y?=w465:bool)
              n380 = Equal?(x=w464, y=5) -> (x = y?=w463:bool)
              n381 = case shown="True" w476 {
                tunnel: w474 -> [_ w488]
                frame False {
                }
                frame True {
                  n382 = Boolean To (0,1)(Boolean=w488) -> (0, 1=w489:i16)
                  n383 = property on="Ring 24" class="Ring (strict)"("Value"=w489) -> ()  [unwired: 2 in, 2 out]
                }
              }
              n384 = case shown="True" w472 {
                tunnel: w474 -> [_ w486]
                frame False {
                }
                frame True {
                  n385 = Boolean To (0,1)(Boolean=w486) -> (0, 1=w487:i16)
                  n386 = property on="Ring 23" class="Ring (strict)"("Value"=w487) -> ()  [unwired: 2 in, 2 out]
                }
              }
              n387 = case shown="True" w467 {
                tunnel: w474 -> [_ w484]
                frame False {
                }
                frame True {
                  n388 = Boolean To (0,1)(Boolean=w484) -> (0, 1=w485:i16)
                  n389 = property on="Ring 22" class="Ring (strict)"("Value"=w485) -> ()  [unwired: 2 in, 2 out]
                }
              }
              n390 = case shown="True" w466 {
                tunnel: w474 -> [_ w482]
                frame False {
                }
                frame True {
                  n391 = Boolean To (0,1)(Boolean=w482) -> (0, 1=w483:i16)
                  n392 = property on="Ring 21" class="Ring (strict)"("Value"=w483) -> ()  [unwired: 2 in, 2 out]
                }
              }
              n393 = case shown="True" w465 {
                tunnel: w474 -> [_ w480]
                frame False {
                }
                frame True {
                  n394 = Boolean To (0,1)(Boolean=w480) -> (0, 1=w481:i16)
                  n395 = property on="Ring 20" class="Ring (strict)"("Value"=w481) -> ()  [unwired: 2 in, 2 out]
                }
              }
              n396 = case shown="True" w463 {
                tunnel: w474 -> [_ w478]
                frame False {
                }
                frame True {
                  n397 = Boolean To (0,1)(Boolean=w478) -> (0, 1=w479:i16)
                  n398 = property on="Ring 19" class="Ring (strict)"("Value"=w479) -> ()  [unwired: 2 in, 2 out]
                }
              }
              n399 = Increment(x=w464) -> (x+1=w477:i32)
              n400 = Not(x=w474) -> (.not. x?=w475:bool)
            }
          }
          n401 = event-data("Discard?"=TRUE) -> ()  [unwired: 4 in, 1 out]
        }
        event "Ring 25", "Ring 26", "Ring 27", "Ring 28", "Ring 29", "Ring 30": Mouse Down? {
          n402 = event-data() -> ("CtlRef"=w501:refnum<vi>)  [unwired: 1 in, 7 out]
          n403 = property class="Ring (strict)"(reference=w501) -> ("Value"=w496:u16)  [unwired: 1 in, 2 out]
          n404 = case shown="2" w496 {
            tunnel: w495 -> [_ w503]
            tunnel: [_ w517] -> w494
            tunnel: w493 -> [_ w515]
            tunnel: [_ w516] -> w492
            frame Default {
            }
            frame 2 {
              n405 = Equal To 0?(x=w503) -> (x = 0?=w514:bool)
              n406 = Equal?(x=w503, y=1) -> (x = y?=w513:bool)
              n407 = Equal?(x=w503, y=2) -> (x = y?=w507:bool)
              n408 = Equal?(x=w503, y=3) -> (x = y?=w506:bool)
              n409 = Equal?(x=w503, y=4) -> (x = y?=w505:bool)
              n410 = Equal?(x=w503, y=5) -> (x = y?=w504:bool)
              n411 = case shown="True" w514 {
                tunnel: w515 -> [_ w528]
                frame False {
                }
                frame True {
                  n412 = Boolean To (0,1)(Boolean=w528) -> (0, 1=w529:i16)
                  n413 = property on="Ring 30" class="Ring (strict)"("Value"=w529) -> ()  [unwired: 2 in, 2 out]
                }
              }
              n414 = case shown="True" w513 {
                tunnel: w515 -> [_ w526]
                frame False {
                }
                frame True {
                  n415 = Boolean To (0,1)(Boolean=w526) -> (0, 1=w527:i16)
                  n416 = property on="Ring 29" class="Ring (strict)"("Value"=w527) -> ()  [unwired: 2 in, 2 out]
                }
              }
              n417 = case shown="True" w507 {
                tunnel: w515 -> [_ w524]
                frame False {
                }
                frame True {
                  n418 = Boolean To (0,1)(Boolean=w524) -> (0, 1=w525:i16)
                  n419 = property on="Ring 28" class="Ring (strict)"("Value"=w525) -> ()  [unwired: 2 in, 2 out]
                }
              }
              n420 = case shown="True" w506 {
                tunnel: w515 -> [_ w522]
                frame False {
                }
                frame True {
                  n421 = Boolean To (0,1)(Boolean=w522) -> (0, 1=w523:i16)
                  n422 = property on="Ring 27" class="Ring (strict)"("Value"=w523) -> ()  [unwired: 2 in, 2 out]
                }
              }
              n423 = case shown="True" w505 {
                tunnel: w515 -> [_ w520]
                frame False {
                }
                frame True {
                  n424 = Boolean To (0,1)(Boolean=w520) -> (0, 1=w521:i16)
                  n425 = property on="Ring 26" class="Ring (strict)"("Value"=w521) -> ()  [unwired: 2 in, 2 out]
                }
              }
              n426 = case shown="True" w504 {
                tunnel: w515 -> [_ w518]
                frame False {
                }
                frame True {
                  n427 = Boolean To (0,1)(Boolean=w518) -> (0, 1=w519:i16)
                  n428 = property on="Ring 25" class="Ring (strict)"("Value"=w519) -> ()  [unwired: 2 in, 2 out]
                }
              }
              n429 = Increment(x=w503) -> (x+1=w517:i32)
              n430 = Not(x=w515) -> (.not. x?=w516:bool)
            }
          }
          n431 = event-data("Discard?"=TRUE) -> ()  [unwired: 4 in, 1 out]
        }
        event "Ring 31", "Ring 32", "Ring 33", "Ring 34", "Ring 35", "Ring 36": Mouse Down? {
          n432 = event-data() -> ("CtlRef"=w537:refnum<vi>)  [unwired: 1 in, 7 out]
          n433 = property class="Ring (strict)"(reference=w537) -> ("Value"=w535:u16)  [unwired: 1 in, 2 out]
          n434 = case shown="2" w535 {
            tunnel: w534 -> [_ w543]
            tunnel: [_ w557] -> w533
            tunnel: w532 -> [_ w555]
            tunnel: [_ w556] -> w531
            frame Default {
            }
            frame 2 {
              n435 = Equal To 0?(x=w543) -> (x = 0?=w554:bool)
              n436 = Equal?(x=w543, y=1) -> (x = y?=w553:bool)
              n437 = Equal?(x=w543, y=2) -> (x = y?=w547:bool)
              n438 = Equal?(x=w543, y=3) -> (x = y?=w546:bool)
              n439 = Equal?(x=w543, y=4) -> (x = y?=w545:bool)
              n440 = Equal?(x=w543, y=5) -> (x = y?=w544:bool)
              n441 = case shown="True" w554 {
                tunnel: w555 -> [_ w568]
                frame False {
                }
                frame True {
                  n442 = Boolean To (0,1)(Boolean=w568) -> (0, 1=w569:i16)
                  n443 = property on="Ring 36" class="Ring (strict)"("Value"=w569) -> ()  [unwired: 2 in, 2 out]
                }
              }
              n444 = case shown="True" w553 {
                tunnel: w555 -> [_ w566]
                frame False {
                }
                frame True {
                  n445 = Boolean To (0,1)(Boolean=w566) -> (0, 1=w567:i16)
                  n446 = property on="Ring 35" class="Ring (strict)"("Value"=w567) -> ()  [unwired: 2 in, 2 out]
                }
              }
              n447 = case shown="True" w547 {
                tunnel: w555 -> [_ w564]
                frame False {
                }
                frame True {
                  n448 = Boolean To (0,1)(Boolean=w564) -> (0, 1=w565:i16)
                  n449 = property on="Ring 34" class="Ring (strict)"("Value"=w565) -> ()  [unwired: 2 in, 2 out]
                }
              }
              n450 = case shown="True" w546 {
                tunnel: w555 -> [_ w562]
                frame False {
                }
                frame True {
                  n451 = Boolean To (0,1)(Boolean=w562) -> (0, 1=w563:i16)
                  n452 = property on="Ring 33" class="Ring (strict)"("Value"=w563) -> ()  [unwired: 2 in, 2 out]
                }
              }
              n453 = case shown="True" w545 {
                tunnel: w555 -> [_ w560]
                frame False {
                }
                frame True {
                  n454 = Boolean To (0,1)(Boolean=w560) -> (0, 1=w561:i16)
                  n455 = property on="Ring 32" class="Ring (strict)"("Value"=w561) -> ()  [unwired: 2 in, 2 out]
                }
              }
              n456 = case shown="True" w544 {
                tunnel: w555 -> [_ w558]
                frame False {
                }
                frame True {
                  n457 = Boolean To (0,1)(Boolean=w558) -> (0, 1=w559:i16)
                  n458 = property on="Ring 31" class="Ring (strict)"("Value"=w559) -> ()  [unwired: 2 in, 2 out]
                }
              }
              n459 = Increment(x=w543) -> (x+1=w557:i32)
              n460 = Not(x=w555) -> (.not. x?=w556:bool)
            }
          }
          n461 = event-data("Discard?"=TRUE) -> ()  [unwired: 4 in, 1 out]
        }
        event "Ring 37", "Ring 38", "Ring 39", "Ring 40", "Ring 41", "Ring 42": Mouse Down? {
          n462 = event-data() -> ("CtlRef"=w582:refnum<vi>)  [unwired: 1 in, 7 out]
          n463 = property class="Ring (strict)"(reference=w582) -> ("Value"=w574:u16)  [unwired: 1 in, 2 out]
          n464 = case shown="2" w574 {
            tunnel: w573 -> [_ w584]
            tunnel: [_ w597] -> w572
            tunnel: w571 -> [_ w595]
            tunnel: [_ w596] -> w570
            frame Default {
            }
            frame 2 {
              n465 = Equal To 0?(x=w584) -> (x = 0?=w594:bool)
              n466 = Equal?(x=w584, y=1.0) -> (x = y?=w592:bool)
              n467 = Equal?(x=w584, y=2.0) -> (x = y?=w587:bool)
              n468 = Equal?(x=w584, y=3.0) -> (x = y?=w586:bool)
              n469 = Equal?(x=w584, y=4.0) -> (x = y?=w585:bool)
              n470 = Equal?(x=w584, y=5.0) -> (x = y?=w583:bool)
              n471 = case shown="True" w594 {
                tunnel: w595 -> [_ w608]
                frame False {
                }
                frame True {
                  n472 = Boolean To (0,1)(Boolean=w608) -> (0, 1=w609:i16)
                  n473 = property on="Ring 42" class="Ring (strict)"("Value"=w609) -> ()  [unwired: 2 in, 2 out]
                }
              }
              n474 = case shown="True" w592 {
                tunnel: w595 -> [_ w606]
                frame False {
                }
                frame True {
                  n475 = Boolean To (0,1)(Boolean=w606) -> (0, 1=w607:i16)
                  n476 = property on="Ring 41" class="Ring (strict)"("Value"=w607) -> ()  [unwired: 2 in, 2 out]
                }
              }
              n477 = case shown="True" w587 {
                tunnel: w595 -> [_ w604]
                frame False {
                }
                frame True {
                  n478 = Boolean To (0,1)(Boolean=w604) -> (0, 1=w605:i16)
                  n479 = property on="Ring 40" class="Ring (strict)"("Value"=w605) -> ()  [unwired: 2 in, 2 out]
                }
              }
              n480 = case shown="True" w586 {
                tunnel: w595 -> [_ w602]
                frame False {
                }
                frame True {
                  n481 = Boolean To (0,1)(Boolean=w602) -> (0, 1=w603:i16)
                  n482 = property on="Ring 39" class="Ring (strict)"("Value"=w603) -> ()  [unwired: 2 in, 2 out]
                }
              }
              n483 = case shown="True" w585 {
                tunnel: w595 -> [_ w600]
                frame False {
                }
                frame True {
                  n484 = Boolean To (0,1)(Boolean=w600) -> (0, 1=w601:i16)
                  n485 = property on="Ring 38" class="Ring (strict)"("Value"=w601) -> ()  [unwired: 2 in, 2 out]
                }
              }
              n486 = case shown="True" w583 {
                tunnel: w595 -> [_ w598]
                frame False {
                }
                frame True {
                  n487 = Boolean To (0,1)(Boolean=w598) -> (0, 1=w599:i16)
                  n488 = property on="Ring 37" class="Ring (strict)"("Value"=w599) -> ()  [unwired: 2 in, 2 out]
                }
              }
              n489 = Increment(x=w584) -> (x+1=w597:i32)
              n490 = Not(x=w595) -> (.not. x?=w596:bool)
            }
          }
          n491 = event-data("Discard?"=TRUE) -> ()  [unwired: 4 in, 1 out]
        }
      }
    }
    n492 = case shown="True" w264 {
      tunnel: w263 -> [_ w269]
      frame False {
      }
      frame True {
        n493 = event shown="[0] \"New Game\": Mouse Up" {
          selector: _ -> [_]
          dyn-events: _ -> [_]
          timeout: _ -> [_]
          tunnel: w269 -> [w270]
          event "New Game": Mouse Up {
            n494 = event-data() -> ()  [unwired: 1 in, 6 out]
            n495 = for {
              tunnel: w270 -> [w272] mode=indexing
              n496 = property class="Ring (strict)"(reference=w272, "Value"=u16 2) -> ()  [unwired: 1 in, 2 out]
            }
          }
        }
      }
    }
  }
